vi "Create Vi.vi"(7 "Vi Type":refnum<class "Vi.lvclass">, 8 "error in":errorcluster, 11 "Vi Info":T1) -> (0 "error out":errorcluster, 3 "Vi out":refnum<class "Vi.lvclass">)   [LabVIEW 2021, in "TAF Proj Document Type.lvlib" / "Vi.lvclass"]
uses:
  <vilib>/Wovalab/AntiDoc/Document Type/Add-ons/LabVIEW TAF Project/Vi/Vi.lvclass
  C:/Program Files (x86)/National Instruments/LabVIEW 2021/vi.lib/Wovalab/AntiDoc/Bloc/Bloc.lvclass
  <vilib>/Wovalab/AntiDoc/Document Type/Add-ons/LabVIEW TAF Project/Vi/Vi Info--cluster.ctl
  <vilib>/picture/picture.llb/imagedata.ctl
  <vilib>/Wovalab/AntiDoc/Bloc/Bloc.lvclass/Bloc.ctl
  <vilib>/Wovalab/AntiDoc/Document Type/Add-ons/LabVIEW TAF Project/Vi/Vi.lvclass/Vi.ctl
  <vilib>/Wovalab/AntiDoc/Bloc/Write Name.vi
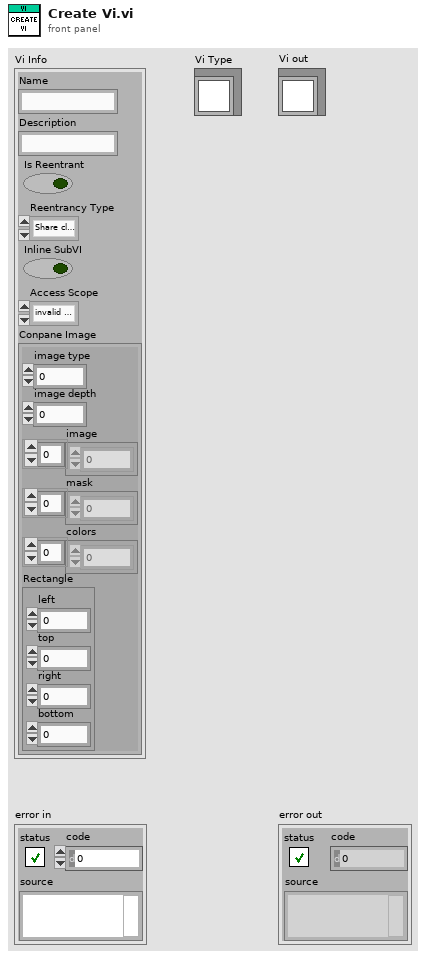
[diagram p1: front panel]
types:
  T1 = typedef "TAF Proj Document Type.lvlib/Vi.lvclass/Vi Info--cluster.ctl" = cluster{"Name":string, "Description":string, "Is Reentrant":bool, "Reentrancy Type":enum16{"Share clones between instances", "Preallocate clone for each instance"}, "Inline SubVI":bool, "Access Scope":enum32{"invalid scope", "public", "private", "protected", "community"}, "Conpane Image":T2}
  T2 = typedef "imagedata.ctl" = cluster{"image type":i32, "image depth":i32, "image":u8[], "mask":u8[], "colors":u32[], "Rectangle":cluster{"left":i16, "top":i16, "right":i16, "bottom":i16}}
  T3 = enum16{"Share clones between instances", "Preallocate clone for each instance"}
  T4 = enum32{"invalid scope", "public", "private", "protected", "community"}
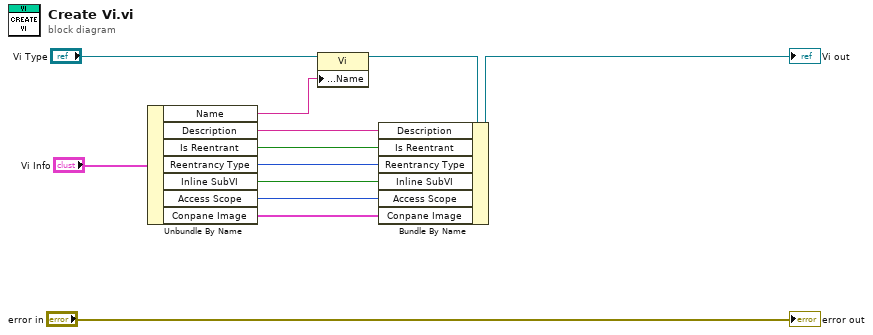
[diagram p0: block diagram]
diagram:
  n1 = Unbundle By Name("Vi Info") -> ("Name"=w3:string, "Description"=w4:string, "Is Reentrant"=w5:bool, "Reentrancy Type"=w6:T3, "Inline SubVI"=w7:bool, "Access Scope"=w8:T4, "Conpane Image"=w9:T2)
  n2 = property class="Vi"(reference="Vi Type", "Accessors:Name"=w3) -> (reference out=w1:refnum<class "Vi.lvclass">)  [unwired: 1 in, 1 out]
  n3 = Bundle By Name(cluster=w1, "Description"=w4, "Is Reentrant"=w5, "Reentrancy Type"=w6, "Inline SubVI"=w7, "Access Scope"=w8, "Conpane Image"=w9) -> (→"Vi out":refnum<class "Vi.lvclass">)
  "error out" <- "error in"
